vi "Find Octave Executable.vi"() -> (1 "Found executable?":bool, 3 "Executable path":path)   [LabVIEW 2020, in "GOLPI library.lvlib"]
doc: "Tries to find GNU Octave executable on disk. Desperate solution to solve BFU issues."
uses:
  GOLPI library.lvlib
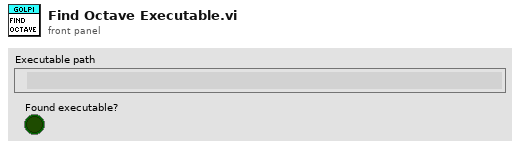
[diagram p1: front panel]
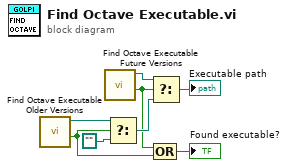
[diagram p0: block diagram]
diagram:
  n1 = call "Find Octave Executable Older Versions.vi"() -> ("Found executable?"=w2:bool, "Executable path"=w6:path)  [unwired: 10 in]
  n2 = call "Find Octave Executable Future Versions.vi"() -> ("Found executable?"=w3:bool, "Executable path"=w8:path)  [unwired: 10 in]
  n3 = Select(t=w6, s=w2, f=path "") -> (s? t:f=w5:path)
  n4 = Select(t=w8, s=w3, f=w5) -> (s? t:f=→"Executable path":path)
  n5 = Compound Arithmetic op=OR(w3, w2) -> (→"Found executable?":bool)
